vi "DMA Read-Windows Host.vi"   [LabVIEW 2012]
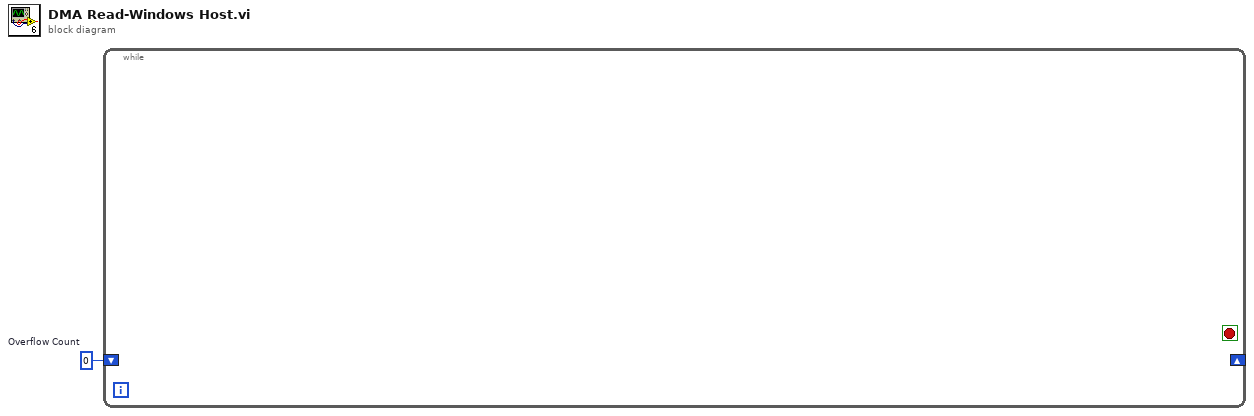
[diagram p0: block diagram]
diagram:
  w1 = u32 0  # Overflow Count
  n1 = while {
    shift-right: _ -> [_]
    shift-left: w1 -> [_]
    stop <- _ stop-if-true
  }
